vi "BARCODE_SEARCH.vi"(8 "error in":errorcluster, 9 "BARCODE_TABLE":string[][](table), 11 "BARCODE_TO_SEARCH":string) -> (0 "error out":errorcluster, 1 "Recipe name":string, 2 "FOUND_ROW":string[](array[string]), 3 "BARCODE_FOUND":bool, 4 "CHL 2":T2, 5 "CHL 1":T3, 6 "CHL 3":T1)   [LabVIEW 2017]
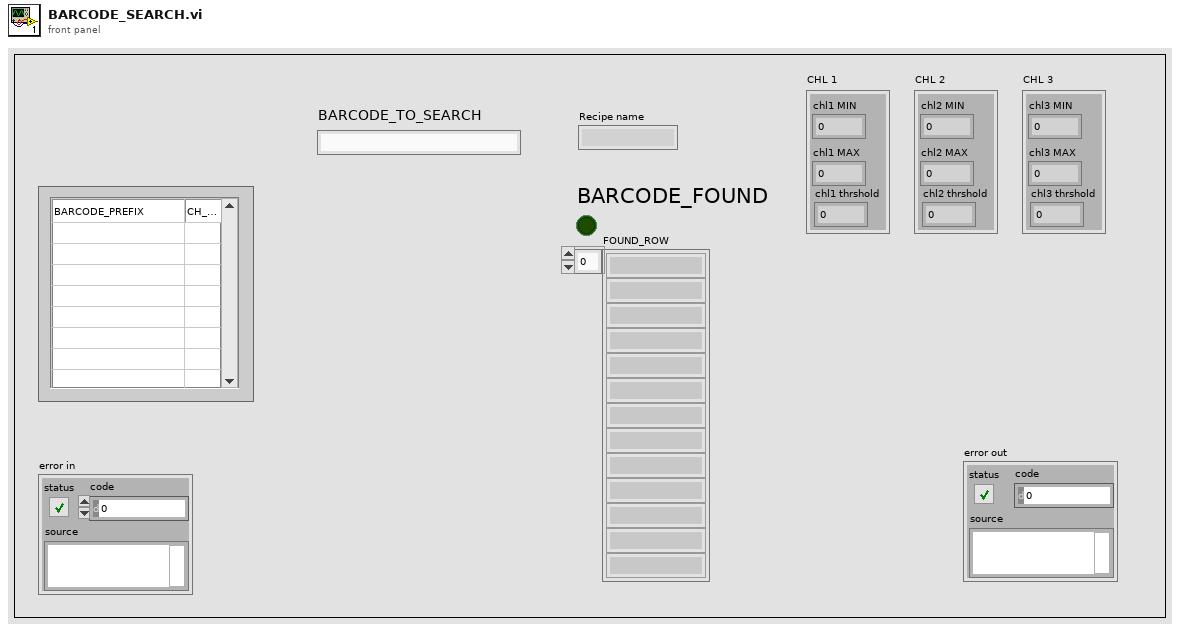
[diagram p1: front panel]
types:
  T1 = cluster{"chl3 MIN":dbl, "chl3 MAX":dbl, "chl3 thrshold":dbl}
  T2 = cluster{"chl2 MIN":dbl, "chl2 MAX":dbl, "chl2 thrshold":dbl}
  T3 = cluster{"chl1 MIN":dbl, "chl1 MAX":dbl, "chl1 thrshold":dbl}
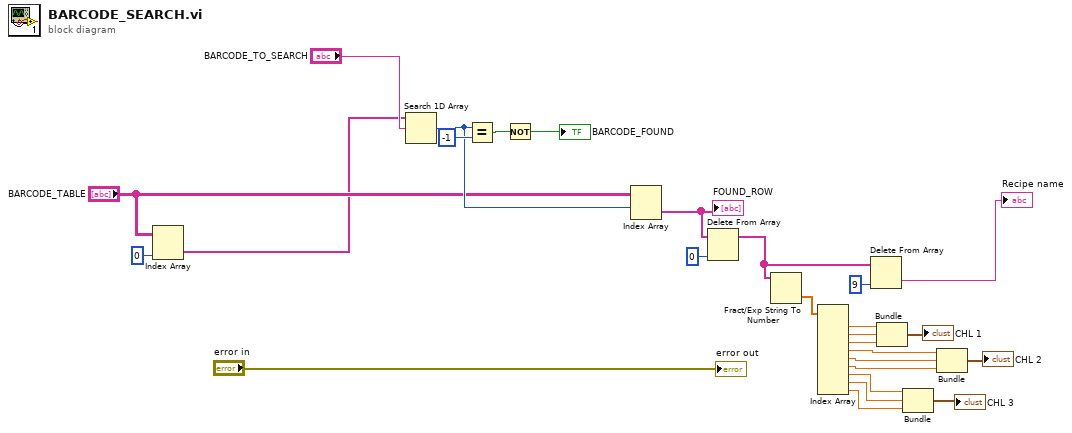
[diagram p0: block diagram]
diagram:
  n1 = Index Array(array="BARCODE_TABLE", index (col)=0 ("disabled index (col)")) -> (element=w4:string[])  [unwired: 1 in]
  n2 = Search 1D Array(1D array=w4, element="BARCODE_TO_SEARCH") -> (index of element=w23:i32)  [unwired: 1 in]
  n3 = Equal?(x=w23, y=-1) -> (x = y?=w26:bool)
  n4 = Not(x=w26) -> (.not. x?=→"BARCODE_FOUND":bool)
  n5 = Index Array(array="BARCODE_TABLE", index (row)=w23) -> (element=w21:string[])  [unwired: 1 in]
  "FOUND_ROW" <- w21
  n6 = Delete From Array(array=w21, index=0) -> (array with subset deleted=w2:string[])  [unwired: 1 in, 1 out]
  n7 = Fract/Exp String To Number(string=w2) -> (number=w19:dbl[])  [unwired: 3 in, 1 out]
  n8 = Index Array(array=w19) -> (element #1=w16:dbl, element #2=w17:dbl, element #3=w18:dbl, element #4=w13:dbl, element #5=w12:dbl, element #6=w11:dbl, element #7=w9:dbl, element #8=w8:dbl, element #9=w7:dbl)  [unwired: 9 in]
  n9 = Delete From Array(array=w2, index=9) -> (deleted portion=→"Recipe name":string)  [unwired: 1 in, 1 out]
  n10 = Bundle(w16, w17, w18) -> (→"CHL 1":cluster{dbl, dbl, dbl})  [unwired: 1 in]
  n11 = Bundle(w9, w8, w7) -> (→"CHL 3":cluster{dbl, dbl, dbl})  [unwired: 1 in]
  n12 = Bundle(w13, w12, w11) -> (→"CHL 2":cluster{dbl, dbl, dbl})  [unwired: 1 in]
  "error out" <- "error in"
